vi "Process Data Reference.vi"(8 "error in (no error)":errorcluster) -> (0 "error out":errorcluster, 3 "process data reference":refnum<data-value>)   [LabVIEW 2015, in "Exposure Process.lvlib"]
uses:
  Exposure Process.lvlib
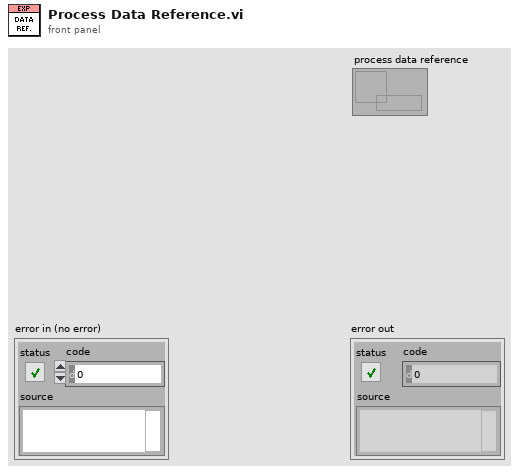
[diagram p1: front panel]
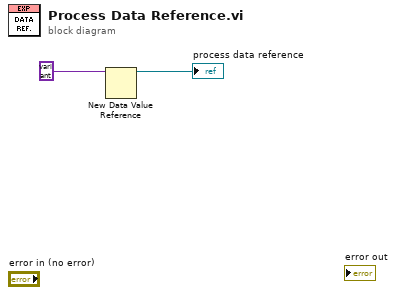
[diagram p0: block diagram]
diagram:
  n1 = New Data Value Reference(data value=variant) -> (data value reference=→"process data reference":refnum<data-value>)  [unwired: 1 in, 1 out]
